vi "QCP_Set_STR.vi"(0 "QCP Data Block In":T1, 1 "QCP Name":string, 2 "Value In":string) -> (7 "QCP Data Block Out":T1)   [LabVIEW 2015]
uses:
  <userlib>/836-Library/System/QCP_Support_Code/QCP_Data_Block.ctl
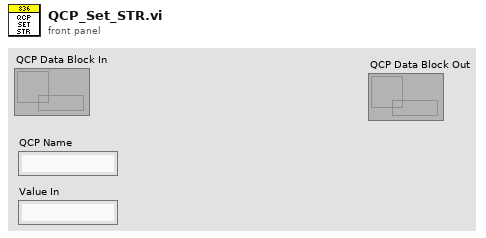
[diagram p1: front panel]
types:
  T1 = typedef "QCP_Data_Block.ctl" = refnum<data-value>
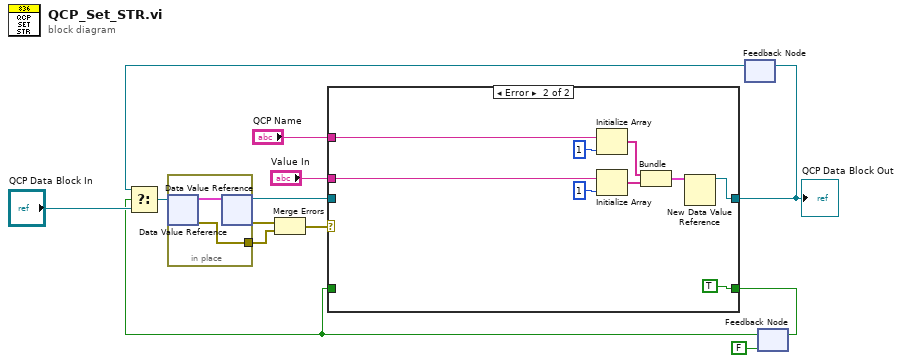
[diagram p0: block diagram]
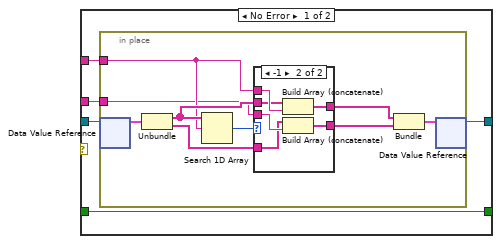
[diagram p2: hidden frame]
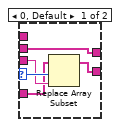
[diagram p3: hidden frame]
diagram:
  n1 = feedback #1() -> (w2:T1)  [unwired: 1 in]
  n2 = feedback #2(FALSE) -> (w3:bool)
  n3 = Select(t=w2, s=w3, f="QCP Data Block In") -> (s? t:f=w4:T1)
  n4 = in-place {
    in-place-border: [w14] -> w12
    n5 = in-place-dvr #3(w4) -> (w15:cluster{string[], string[]}, w14:errorcluster)
    n6 = in-place-dvr #3(w15) -> (w10:T1, w13:errorcluster)
  }
  n7 = Merge Errors(w13, w12) -> (w11:errorcluster)
  n8 = case shown="Error" w11 {
    tunnel: [w20 w43] -> w8
    tunnel: w10 -> [w19 _]
    tunnel: "QCP Name" -> [w18 w49]
    tunnel: [w17 TRUE] -> w7
    tunnel: w3 -> [w17 _]
    tunnel: "Value In" -> [w16 w41]
    frame No Error {
      n9 = in-place {
        in-place-border: w18 -> [w22]
        in-place-border: w16 -> [w21]
        n10 = in-place-dvr #4(w19) -> (w29:cluster{string[], string[]})  [unwired: 1 out]
        n11 = Unbundle(w29) -> (w25:string[], w26:string[])
        n12 = Search 1D Array(1D array=w25, element=w22) -> (index of element=w27:i32)  [unwired: 1 out]
        n13 = case shown="-1" w27 {
          selector: w27 -> [w34 _]
          tunnel: w22 -> [_ w40]
          tunnel: [w31 w39] -> w24
          tunnel: w21 -> [w33 w38]
          tunnel: [w32 w37] -> w23
          tunnel: w26 -> [w30 w36]
          tunnel: w25 -> [w31 w35]
          frame 0, Default {
            n14 = Replace Array Subset(array=w30, new element=w33, index=w34) -> (w32:string[])
          }
          frame -1 {
            n15 = Build Array (concatenate)(w35, w40) -> (w39:string[])
            n16 = Build Array (concatenate)(w36, w38) -> (w37:string[])
          }
        }
        n17 = Bundle(w24, w23) -> (w28:cluster{string[], string[]})  [unwired: 1 in]
        n18 = in-place-dvr #4(w28) -> (w20:T1)  [unwired: 1 out]
      }
    }
    frame Error {
      n19 = Initialize Array(w49, 1 ("dimension size")) -> (w45:string[])
      n20 = Initialize Array(w41, 1 ("dimension size")) -> (w46:string[])
      n21 = Bundle(w45, w46) -> (w44:cluster{string[], string[]})  [unwired: 1 in]
      n22 = New Data Value Reference(data value=w44) -> (data value reference=w43:refnum<data-value>)  [unwired: 1 in, 1 out]
    }
  }
  "QCP Data Block Out" <- w8
  n23 = feedback-in #1(w8) -> ()
  n24 = feedback-in #2(w7) -> ()
